vi "Sub_ProhibitedString.vi"(11 "入力文字列":string) -> (2 "一致した文字位置":i32, 3 "一致?":bool)   [LabVIEW 2018]
uses:
  <vilib>/regexp/Match Regular Expression.xnode
panel:
  # "<機能>\n　禁止文字列のチェックをする。\n　禁止文字列は定数で定義"
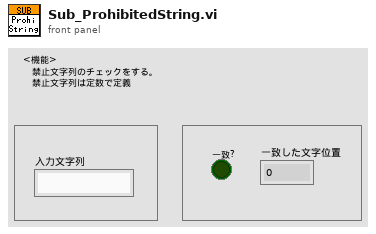
[diagram p1: front panel]
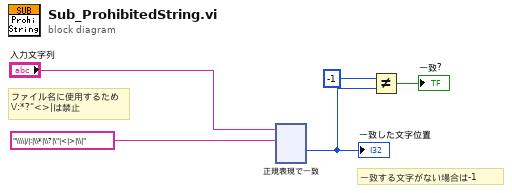
[diagram p0: block diagram]
diagram:
  # "一致する文字がない場合は-1"
  # "ファイル名に使用するため\n\\/:*?\"<>|は禁止"
  n1 = xnode "正規表現で一致"("入力文字列"="入力文字列", "正規表現"="\\\\|/|:|\\*|\\?|\"|<|>|\\|") -> ("一致後オフセット"=w3:i32)  [unwired: 4 in, 4 out]
  "一致した文字位置" <- w3
  n2 = Not Equal?(x=-1, y=w3) -> (x != y?=→"一致?":bool)
